vi "j_MotorExecute.vi"(5 "MoveChamber?":bool, 6 "Axis Motor Settings":T1={"Joyst Min Signal"=50.0, "Joyst Max Signal"=50.0, "Vmax (mm/s)"=0.3, "Acc (mm/s/s)"=0.5, "+ JoystDirection"=0, "- JoystDirection"=0} {"Acc (mm/s/s)" format="%#.3f"; "Vmax (mm/s)" format="%#.3f"}, 7 "Error In":errorcluster, 8 "JoystRelPos":i32, 9 "Motor's Old Direction":i32, 10 "Motor Reference In":refnum<k7>) -> (0 "Error Out":errorcluster, 1 "Motor Position (mm)":sgl, 2 "Motor's New Direction":i32, 3 "Motor Reference":refnum<k7>, 4 "Motor Velocity (mm/s)":sgl)   [LabVIEW 2014]
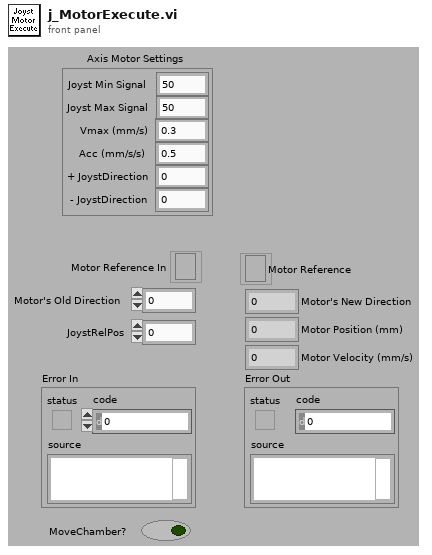
[diagram p1: front panel]
types:
  T1 = cluster{"Joyst Min Signal":dbl, "Joyst Max Signal":dbl, "Vmax (mm/s)":sgl, "Acc (mm/s/s)":sgl, "+ JoystDirection":i32, "- JoystDirection":i32}
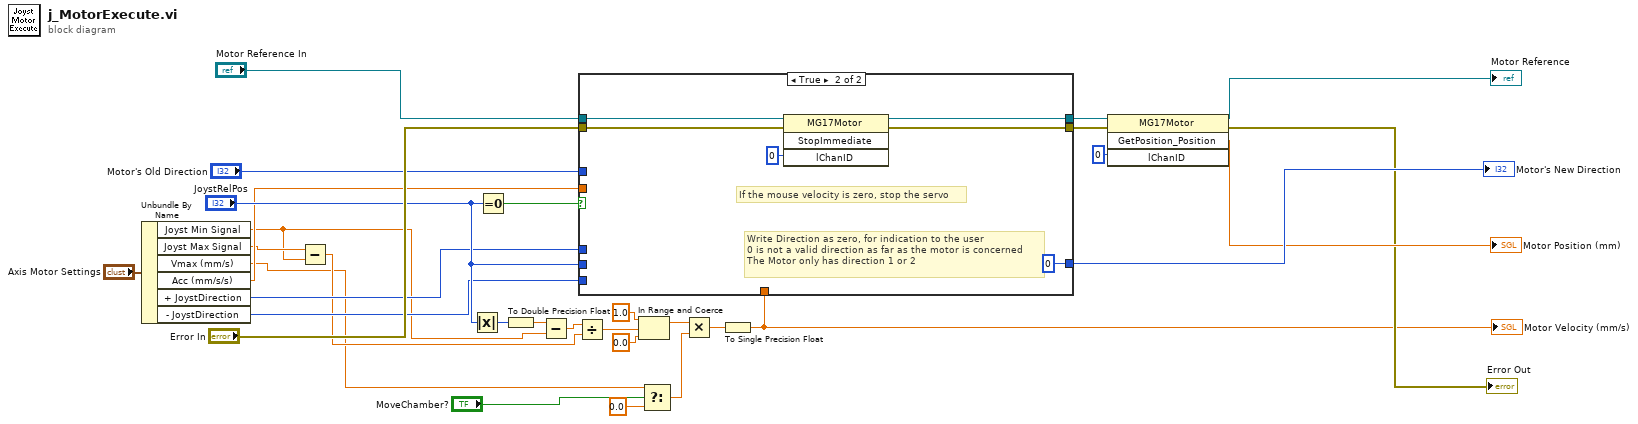
[diagram p0: block diagram]
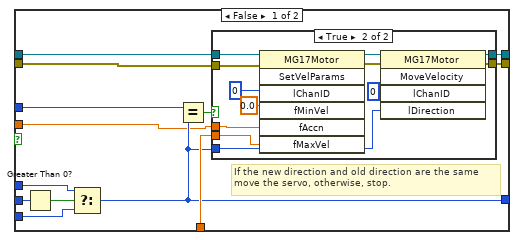
[diagram p2: hidden frame]
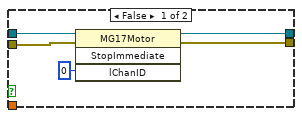
[diagram p3: hidden frame]
diagram:
  n1 = Unbundle By Name("Axis Motor Settings") -> ("Joyst Min Signal"=w3:dbl, "Joyst Max Signal"=w4:dbl, "Vmax (mm/s)"=w1:sgl, "Acc (mm/s/s)"=w7:sgl, "+ JoystDirection"=w9:i32, "- JoystDirection"=w8:i32)
  n2 = Subtract(x=w4, y=w3) -> (x-y=w2:dbl)
  n3 = Absolute Value(x="JoystRelPos") -> (abs(x)=w11:i32)
  n4 = Equal To 0?(x="JoystRelPos") -> (x = 0?=w18:bool)
  n5 = To Double Precision Float(number=w11) -> (double precision float=w6:dbl)
  n6 = Subtract(x=w6, y=w3) -> (x-y=w5:dbl)
  n7 = Divide(x=w5, y=w2) -> (x/y=w13:dbl)
  n8 = In Range and Coerce(upper limit=1.0, x=w13, lower limit=0.0) -> (coerced(x)=w15:dbl)  [unwired: 1 out]
  n9 = Select(t=w1, s="MoveChamber?", f=0.0) -> (s? t:f=w16:dbl)
  n10 = Multiply(x=w15, y=w16) -> (x*y=w20:dbl)
  n11 = To Single Precision Float(number=w20) -> (single precision float=w22:sgl)
  "Motor Velocity (mm/s)" <- w22
  n12 = case shown="True" w18 {
    tunnel: [w37 0 ("f")] -> w31
    tunnel: "JoystRelPos" -> [w45 _]
    tunnel: w22 -> [w43 _]
    tunnel: [w42 w65] -> w25
    tunnel: [w41 w64] -> w26
    tunnel: "Motor Reference In" -> [w40 w67]
    tunnel: "Error In" -> [w39 w66]
    tunnel: "Motor's Old Direction" -> [w38 _]
    tunnel: w9 -> [w35 _]
    tunnel: w8 -> [w34 _]
    tunnel: w7 -> [w33 _]
    frame False {
      # "If the new direction and old direction are the same\nmove the servo, otherwise, stop."
      n13 = Greater Than 0?(x=w45) -> (x > 0?=w44:bool)
      n14 = Select(t=w35, s=w44, f=w34) -> (s? t:f=w37:i32)
      n15 = Equal?(x=w38, y=w37) -> (x = y?=w36:bool)
      n16 = case shown="True" w36 {
        tunnel: w43 -> [_ w52]
        tunnel: [w47 w57] -> w42
        tunnel: [w46 w56] -> w41
        tunnel: w40 -> [w49 w55]
        tunnel: w39 -> [w48 w54]
        tunnel: w37 -> [_ w53]
        tunnel: w33 -> [_ w51]
        frame False {
          n17 = invoke class="MG17Motor" method="StopImmediate"(reference=w49, error in=w48, "lChanID"=0) -> (reference out=w47:refnum<k7>, error out=w46:errorcluster)  [unwired: 1 in, 2 out]
        }
        frame True {
          n18 = invoke class="MG17Motor" method="SetVelParams"(reference=w55, error in=w54, "lChanID"=0, "fMinVel"=sgl 0.0, "fAccn"=w51, "fMaxVel"=w52) -> (reference out=w60:refnum<k7>, error out=w59:errorcluster)  [unwired: 1 in, 5 out]
          n19 = invoke class="MG17Motor" method="MoveVelocity"(reference=w60, error in=w59, "lChanID"=0, "lDirection"=w53) -> (reference out=w57:refnum<k7>, error out=w56:errorcluster)  [unwired: 1 in, 3 out]
        }
      }
    }
    frame True {
      # "Write Direction as zero, for indication to the user\n0 is not a valid direction as far as the motor is concerned\nThe Motor only has direction 1 or 2"
      # "If the mouse velocity is zero, stop the servo"
      n20 = invoke class="MG17Motor" method="StopImmediate"(reference=w67, error in=w66, "lChanID"=0) -> (reference out=w65:refnum<k7>, error out=w64:errorcluster)  [unwired: 1 in, 2 out]
    }
  }
  "Motor's New Direction" <- w31
  n21 = invoke class="MG17Motor" method="GetPosition_Position"(reference=w25, error in=w26, "lChanID"=0) -> (reference out=→"Motor Reference":refnum<k7>, error out=→"Error Out":errorcluster, "GetPosition_Position"=→"Motor Position (mm)":sgl)  [unwired: 1 in, 1 out]
